vi "Init.vi"(8 "error in (no error)":errorcluster, 11 "Data in":refnum<class "OnChange_Boolean.lvclass">) -> (0 "error out":errorcluster, 3 "Data out":refnum<class "OnChange_Boolean.lvclass">)   [LabVIEW 2021, in "OnChange_Boolean.lvclass"]
doc: "Abstract Data Classes 2.1.1.13\nTim Streeter - TSA\nCopyright (c) 2025, TSA"
uses:
  OnChange_Boolean.lvclass
  C:/Program Files (x86)/National Instruments/LabVIEW 2021/vi.lib/TSA/Abstract Data Classes/Abs_Types/Value/Abs_Value.lvclass
  OnChange_Boolean.lvclass/OnChange_Boolean.ctl
  Properties/Read Data Type.vi
  Properties/Write Data Type.vi
  <vilib>/TSA/Abstract Data Classes/Abs_Types/Boolean/Abs_Boolean.lvclass
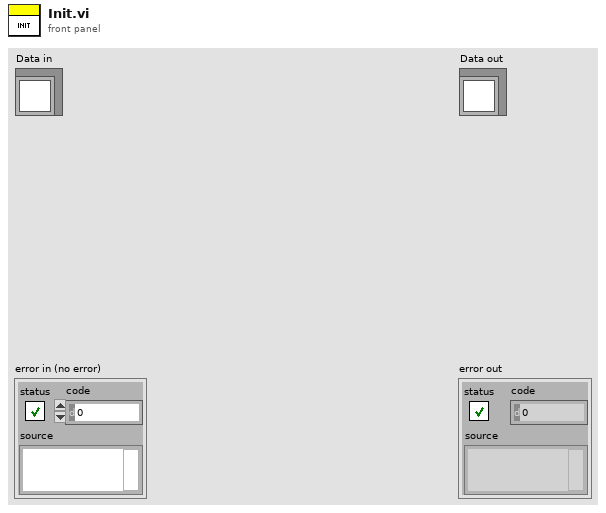
[diagram p1: front panel]
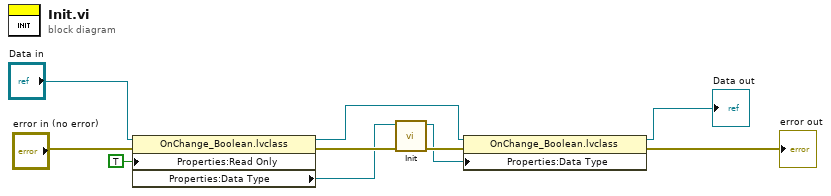
[diagram p0: block diagram]
diagram:
  n1 = property class="OnChange_Boolean.lvclass"(reference="Data in", error in="error in (no error)", "Properties:Read Only"=TRUE ("Read Only")) -> (reference out=w5:refnum<class "OnChange_Boolean.lvclass">, error out=w7:errorcluster, "Properties:Data Type"=w4:refnum<class "Abs_Boolean.lvclass">)
  n2 = call-dynamic "Init.vi"("error in (no error)"=w7, "Data in"=w4) -> ("error out"=w6:errorcluster, "Data out"=w3:refnum<class "Abs_Boolean.lvclass">)  [unwired: 8 in]
  n3 = property class="OnChange_Boolean.lvclass"(reference=w5, error in=w6, "Properties:Data Type"=w3) -> (reference out=→"Data out":refnum<class "OnChange_Boolean.lvclass">, error out=→"error out":errorcluster)
